vi "XYZ stage handler_coMD.vi"() -> ()   [LabVIEW 2012]
doc: "SciScan 1.2 160622"
uses:
  <vilib>/Analysis/coordinate.llb/Euler Rotation Order.ctl
  <vilib>/Utility/VariantDataType/Type.ctl
  GFG/GFGnumericGet.vi
  GFG/GFGbooleanGet.vi
  <vilib>/Analysis/coordinate.llb/3D Cartesian Coordinate Rotation (Euler) (Scalar).vi
  GFG/GFGfpRefGet.vi
  GFG/GFG library.lvlib
  <vilib>/Analysis/NI_AALPro.lvlib
  <vilib>/Utility/VariantDataType/VariantType.lvlib
panel:
  out "error out 2":errorcluster
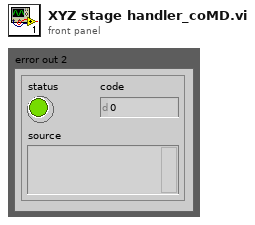
[diagram p1: front panel]
types:
  T1 = enum16{"none", "quit", "Press", "Long Press", "Long Press finished", "Short Press finished"}
  T2 = cluster{"WaveformChartRef":refnum<vi>, "DigitalRef":refnum<vi>, "ArrayRef":refnum<vi>, "TabControlRef":refnum<vi>, "EnumRef":refnum<vi>, "RingRef":refnum<vi>, "BooleanRef":refnum<vi>, "KnobRef":refnum<vi>, "SlideRef":refnum<vi>, "PathRef":refnum<vi>, "StringRef":refnum<vi>, "ComboBox":refnum<vi>, "WaveformGraphRef":refnum<vi>}
  T3 = cluster{"Xoffset":dbl, "Yoffset":dbl, "Zoffset":dbl}
  T4 = cluster{"moveXabs":dbl, "moveYabs":dbl, "moveZabs":dbl}
  T5 = cluster{"new pos X":dbl, "new pos Y":dbl, "new pos Z":dbl}
  T6 = typedef "NI_AALPro.lvlib/Euler Rotation Order.ctl" = u16
  T7 = cluster{"Numeric":dbl, "Numeric":dbl, "Numeric":dbl}
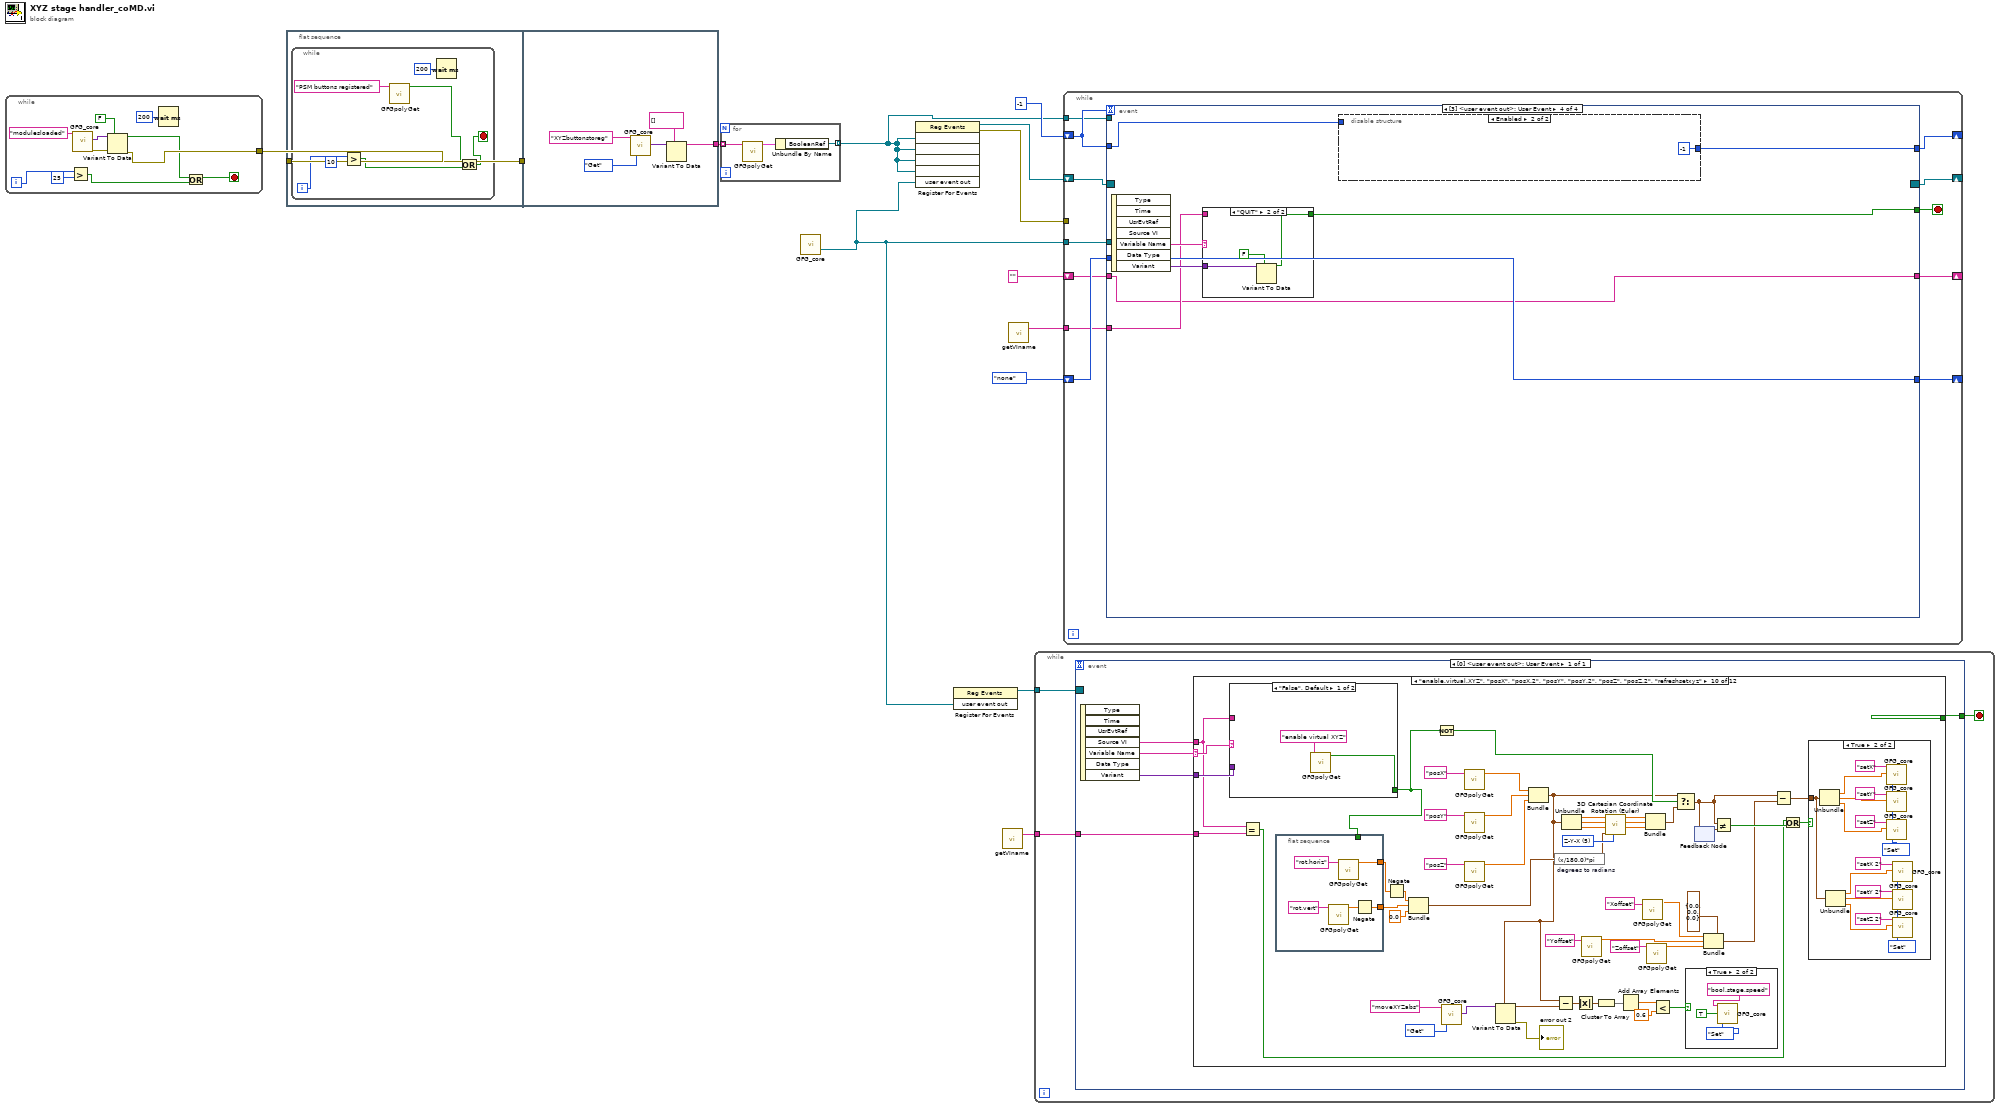
[diagram p0: block diagram]
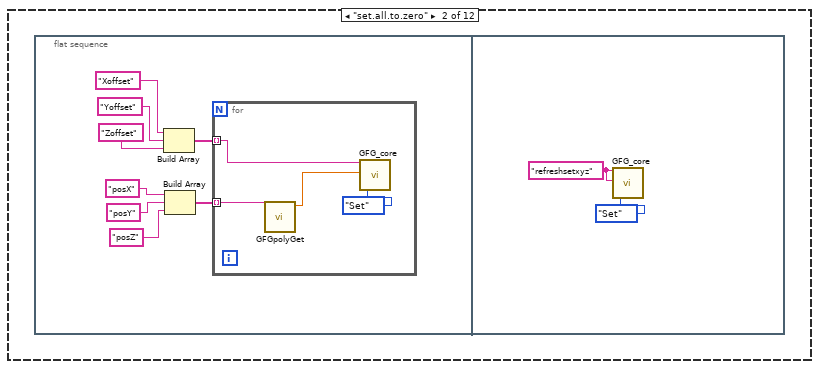
[diagram p3: hidden frame]
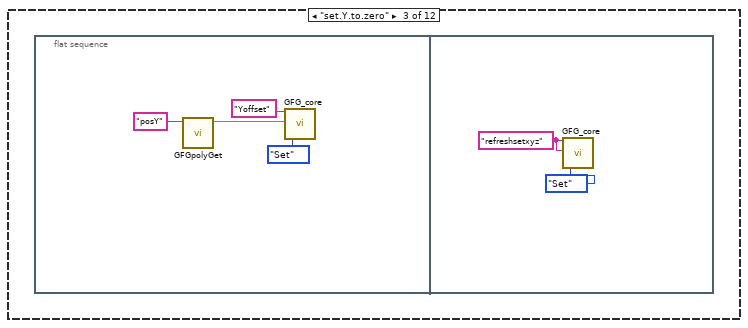
[diagram p4: hidden frame]
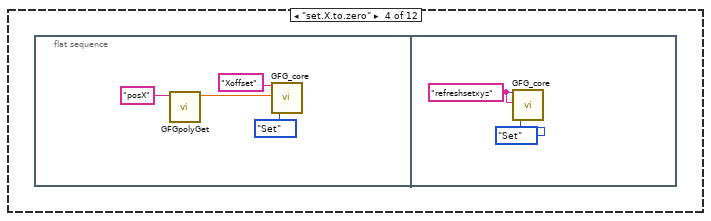
[diagram p5: hidden frame]
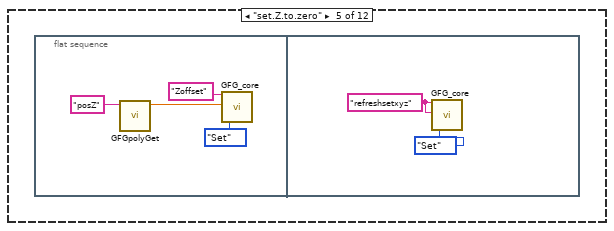
[diagram p6: hidden frame]
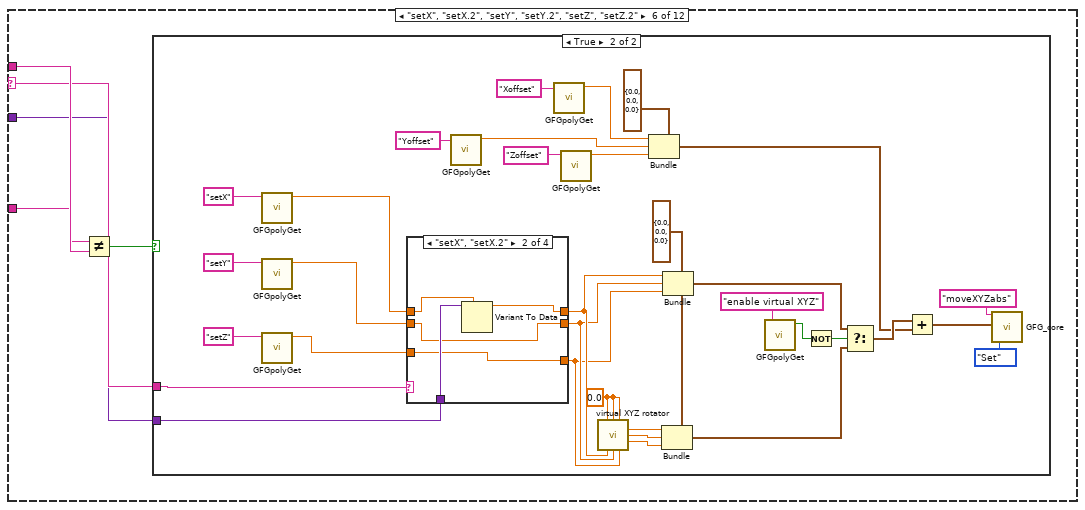
[diagram p7: hidden frame]
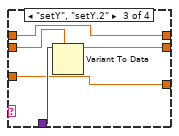
[diagram p10: hidden frame]
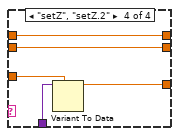
[diagram p11: hidden frame]
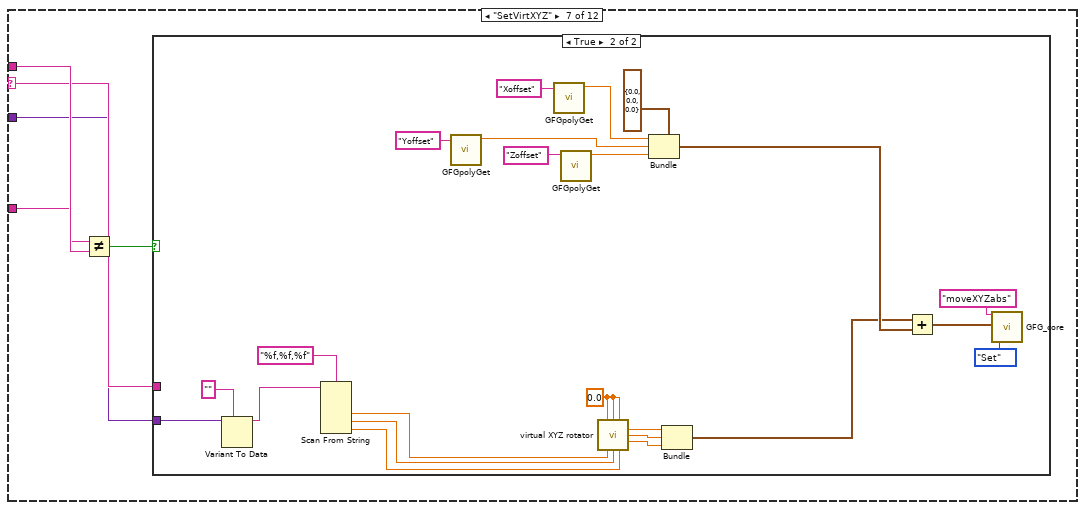
[diagram p12: hidden frame]
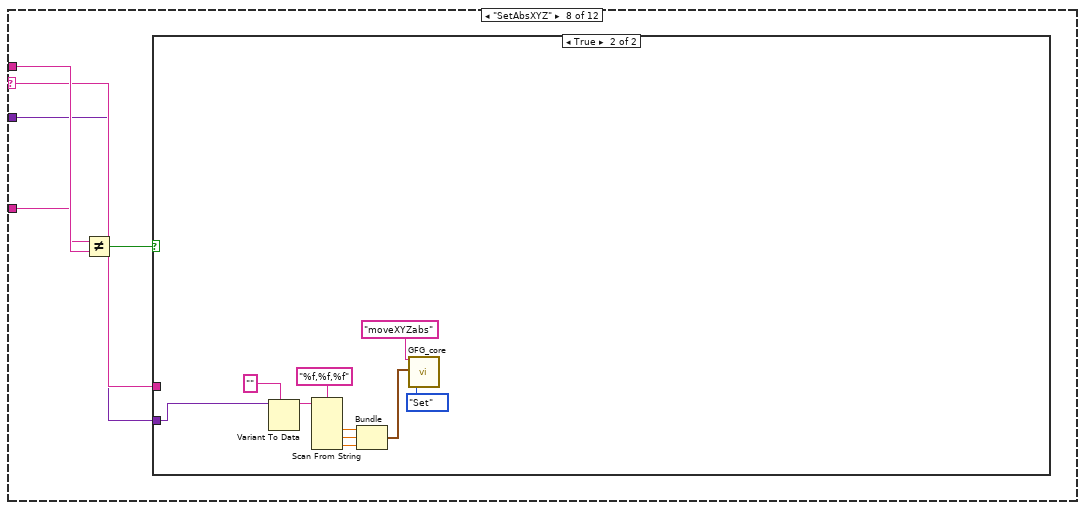
[diagram p14: hidden frame]
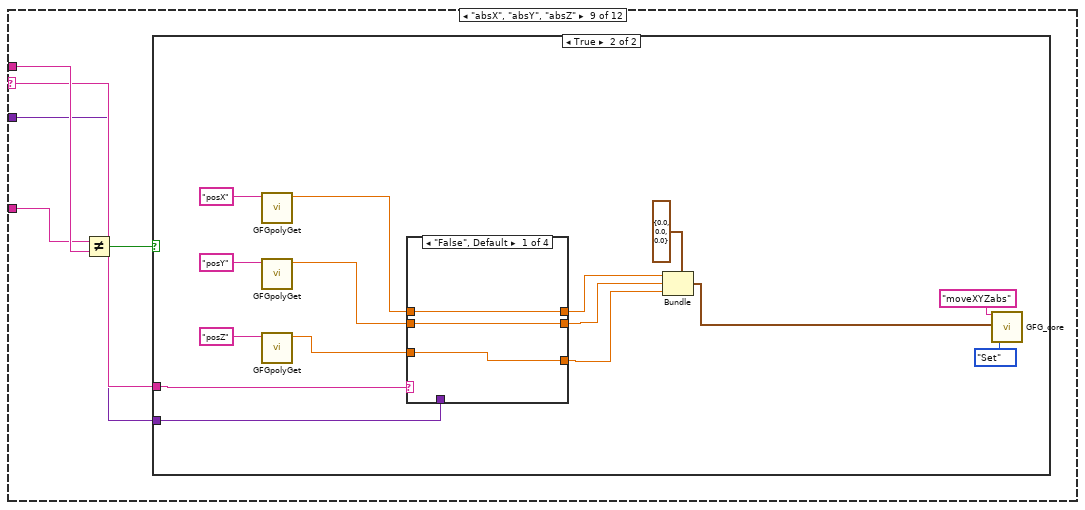
[diagram p16: hidden frame]
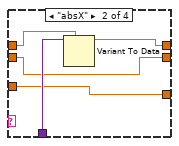
[diagram p18: hidden frame]
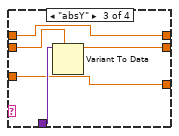
[diagram p19: hidden frame]
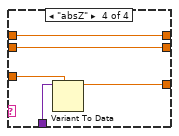
[diagram p20: hidden frame]
diagram:
  n1 = while {
    tunnel: [w19] -> w6
    i -> [w16]
    stop <- w17 stop-if-true
    n2 = Greater?(x=w16, y=25) -> (0:w14:bool)
    n3 = call "GFG_core.vi"("Variable Name in"="modulesloaded") -> ("Variant Out"=w20:variant, "error out"=w22:errorcluster)  [unwired: 12 in, 5 out]
    n4 = Variant To Data(error in=w22, type=FALSE, Variant=w20) -> (data=w18:bool, error out=w19:errorcluster)
    n5 = Wait (ms)(milliseconds to wait=u32 200) -> ()  [unwired: 1 out]
    n6 = Or(x=w18, y=w14) -> (x .or. y?=w17:bool)
  }
  n7 = flat-sequence {
    tunnel: w6 -> [w25]
    tunnel: [w25] -> w5
    tunnel: [w37] -> w7
    tunnel: w5 -> [_]
    frame #0 {
      n8 = while {
        i -> [w28]
        stop <- w26 stop-if-true
        n9 = Greater?(x=w28, y=10) -> (0:w30:bool)
        n10 = call-poly "GFGpolyGet.vi"("Variable Name in"="PSM buttons registered") -> ("Boolean Value OUT"=w27:bool)  [unwired: 9 in, 1 out]
        n11 = Wait (ms)(milliseconds to wait=u32 200) -> ()  [unwired: 1 out]
        n12 = Or(x=w27, y=w30) -> (x .or. y?=w26:bool)
      }
    }
    frame #1 {
      n13 = call "GFG_core.vi"("Variable Name in"="XYZbuttonstoreg", "Action"=enum16{"Init", "Set", "Get"}."Get") -> ("Variant Out"=w33:variant)  [unwired: 11 in, 6 out]
      n14 = Variant To Data(type=string[] [], Variant=w33) -> (data=w37:string[])  [unwired: 1 in, 1 out]
    }
  }
  n15 = for {
    tunnel: w7 -> [w39] mode=indexing
    tunnel: [w38] -> w4 mode=indexing
    n16 = call-poly "GFGpolyGet.vi"("Variable Name in"=w39) -> ("output cluster"=w40:T2)  [unwired: 9 in, 1 out]
    n17 = Unbundle By Name(w40) -> ("BooleanRef"=w38:refnum<vi>)
  }
  n18 = call "GFG_core.vi"() -> ("user event out"=w3:refnum<user-event>)  [unwired: 13 in, 6 out]
  n19 = register-events(w4, w4, w4, w4, w3) -> (reference out=w8:refnum<event-registration>, error out=w9:errorcluster)  [unwired: 2 in]
  n20 = register-events(w3) -> (reference out=w1:refnum<event-registration>)  [unwired: 2 in, 1 out]
  n21 = call "getVIname.vi"() -> ("VI name"=w2:string)  [unwired: 19 in]
  n22 = call "getVIname.vi"() -> ("VI name"=w10:string)  [unwired: 19 in]
  n23 = while {
    tunnel: w2 -> [w42]
    tunnel: w1 -> [w41]
    stop <- w43 stop-if-true
    n24 = event shown="[0] <user event out>: User Event" {
      selector: w41 -> [_]
      dyn-events: _ -> [_]
      timeout: _ -> [_]
      tunnel: [w46] -> w43
      tunnel: w42 -> [w44]
      event User Event {
        n25 = event-data() -> ("Source VI"=w45:string, "Variable Name"=w47:string, "Variant"=w48:variant)  [unwired: 1 in, 4 out]
        n26 = case shown="\"enable.virtual.XYZ\", \"posX\", \"posX.2\", \"posY\", \"posY.2\", \"posZ\", \"posZ.2\", \"refreshsetxyz\"" w47 {
          selector: w47 -> [_ _ _ _ _ w82 w138 w166 w181 w269 _ w308]
          tunnel: [_ _ _ _ _ _ _ _ _ _ w302 _] -> w46
          tunnel: w48 -> [_ _ _ _ _ w81 w137 w165 w180 w268 w304 _]
          tunnel: w45 -> [_ _ _ _ _ w85 w141 w169 w184 w218 _ _]
          tunnel: w44 -> [_ _ _ _ _ w84 w140 w168 w183 w220 _ _]
          frame "False", Default {
          }
          frame "set.all.to.zero" {
            n27 = flat-sequence {
              frame #0 {
                n28 = Build Array("Xoffset" ("Variable Name in"), "Yoffset" ("Variable Name in"), "Zoffset" ("Variable Name in")) -> (w56:string[])
                n29 = Build Array("posX" ("Variable Name in"), "posY" ("Variable Name in"), "posZ" ("Variable Name in")) -> (w52:string[])
                n30 = for {
                  tunnel: w52 -> [w59] mode=indexing
                  tunnel: w56 -> [w57] mode=indexing
                  n31 = call-poly "GFGpolyGet.vi"("Variable Name in"=w59) -> ("Numeric"=w58:dbl)  [unwired: 8 in, 2 out]
                  n32 = call "GFG_core.vi"("Variable Name in"=w57, "Variant in"=w58, "Action"=enum16{"Init", "Set", "Get"}."Set") -> ()  [unwired: 10 in, 7 out]
                }
              }
              frame #1 {
                w61 = "refreshsetxyz" ("Variable Name in")
                n33 = call "GFG_core.vi"("Variable Name in"=w61, "Variant in"=w61, "Action"=enum16{"Init", "Set", "Get"}."Set") -> ()  [unwired: 10 in, 7 out]
              }
            }
          }
          frame "set.Y.to.zero" {
            n34 = flat-sequence {
              frame #0 {
                n35 = call-poly "GFGpolyGet.vi"("Variable Name in"="posY") -> ("Numeric"=w64:dbl)  [unwired: 8 in, 2 out]
                n36 = call "GFG_core.vi"("Variable Name in"="Yoffset", "Variant in"=w64, "Action"=enum16{"Init", "Set", "Get"}."Set") -> ()  [unwired: 10 in, 7 out]
              }
              frame #1 {
                w67 = "refreshsetxyz" ("Variable Name in")
                n37 = call "GFG_core.vi"("Variable Name in"=w67, "Variant in"=w67, "Action"=enum16{"Init", "Set", "Get"}."Set") -> ()  [unwired: 10 in, 7 out]
              }
            }
          }
          frame "set.X.to.zero" {
            n38 = flat-sequence {
              frame #0 {
                n39 = call-poly "GFGpolyGet.vi"("Variable Name in"="posX") -> ("Numeric"=w70:dbl)  [unwired: 8 in, 2 out]
                n40 = call "GFG_core.vi"("Variable Name in"="Xoffset", "Variant in"=w70, "Action"=enum16{"Init", "Set", "Get"}."Set") -> ()  [unwired: 10 in, 7 out]
              }
              frame #1 {
                w73 = "refreshsetxyz" ("Variable Name in")
                n41 = call "GFG_core.vi"("Variable Name in"=w73, "Variant in"=w73, "Action"=enum16{"Init", "Set", "Get"}."Set") -> ()  [unwired: 10 in, 7 out]
              }
            }
          }
          frame "set.Z.to.zero" {
            n42 = flat-sequence {
              frame #0 {
                n43 = call-poly "GFGpolyGet.vi"("Variable Name in"="posZ") -> ("Numeric"=w76:dbl)  [unwired: 8 in, 2 out]
                n44 = call "GFG_core.vi"("Variable Name in"="Zoffset", "Variant in"=w76, "Action"=enum16{"Init", "Set", "Get"}."Set") -> ()  [unwired: 10 in, 7 out]
              }
              frame #1 {
                w79 = "refreshsetxyz" ("Variable Name in")
                n45 = call "GFG_core.vi"("Variable Name in"=w79, "Variant in"=w79, "Action"=enum16{"Init", "Set", "Get"}."Set") -> ()  [unwired: 10 in, 7 out]
              }
            }
          }
          frame "setX", "setX.2", "setY", "setY.2", "setZ", "setZ.2" {
            n46 = Not Equal?(x=w84, y=w85) -> (x != y?=w83:bool)
            n47 = case shown="True" w83 {
              tunnel: w82 -> [_ w112]
              tunnel: w81 -> [_ w111]
              frame False {
              }
              frame True {
                w101 = 0.0 ("current pos X")
                w106 = T4 {"moveXabs"=0.0, "moveYabs"=0.0, "moveZabs"=0.0} ("output cluster")
                n48 = call-poly "GFGpolyGet.vi"("Variable Name in"="setX") -> ("Numeric"=w117:dbl)  [unwired: 8 in, 2 out]
                n49 = call-poly "GFGpolyGet.vi"("Variable Name in"="setY") -> ("Numeric"=w116:dbl)  [unwired: 8 in, 2 out]
                n50 = call-poly "GFGpolyGet.vi"("Variable Name in"="setZ") -> ("Numeric"=w118:dbl)  [unwired: 8 in, 2 out]
                n51 = case shown="\"setX\", \"setX.2\"" w112 {
                  tunnel: w116 -> [w120 w125 w128 w134]
                  tunnel: w117 -> [w121 w122 w129 w135]
                  tunnel: w118 -> [w119 w123 w130 w133]
                  tunnel: w111 -> [_ w126 w131 w136]
                  tunnel: [w120 w125 w127 w134] -> w96
                  tunnel: [w121 w124 w129 w135] -> w97
                  tunnel: [w119 w123 w130 w132] -> w95
                  frame "False", Default {
                  }
                  frame "setX", "setX.2" {
                    n52 = Variant To Data(type=w122, Variant=w126) -> (data=w124:dbl)  [unwired: 1 in, 1 out]
                  }
                  frame "setY", "setY.2" {
                    n53 = Variant To Data(type=w128, Variant=w131) -> (data=w127:dbl)  [unwired: 1 in, 1 out]
                  }
                  frame "setZ", "setZ.2" {
                    n54 = Variant To Data(type=w133, Variant=w136) -> (data=w132:dbl)  [unwired: 1 in, 1 out]
                  }
                }
                n55 = call-poly "GFGpolyGet.vi"("Variable Name in"="Yoffset") -> ("Numeric"=w88:dbl)  [unwired: 8 in, 2 out]
                n56 = call-poly "GFGpolyGet.vi"("Variable Name in"="Xoffset") -> ("Numeric"=w89:dbl)  [unwired: 8 in, 2 out]
                n57 = call-poly "GFGpolyGet.vi"("Variable Name in"="Zoffset") -> ("Numeric"=w87:dbl)  [unwired: 8 in, 2 out]
                n58 = call "virtual XYZ rotator.vi"("current pos X"=w101, "current pos Y"=w101, "current pos Z"=w101, "virtual X relative"=w97, "virtual Y relative"=w96, "virtual Z relative"=w95) -> ("new pos X"=w109:dbl, "new pos Y"=w108:dbl, "new pos Z"=w107:dbl)  [unwired: 7 in]
                n59 = Bundle(cluster=T3 {"Xoffset"=0.0, "Yoffset"=0.0, "Zoffset"=0.0} ("output cluster"), "Xoffset"=w89, "Yoffset"=w88, "Zoffset"=w87) -> (w86:T3)
                n60 = Bundle(cluster=w106, "moveXabs"=w109, "moveYabs"=w108, "moveZabs"=w107) -> (w104:T4)
                n61 = Bundle(cluster=w106, "moveXabs"=w97, "moveYabs"=w96, "moveZabs"=w95) -> (w105:T4)
                n62 = call-poly "GFGpolyGet.vi"("Variable Name in"="enable virtual XYZ") -> ("Boolean Value OUT"=w103:bool)  [unwired: 9 in, 1 out]
                n63 = Not(x=w103) -> (.not. x?=w102:bool)
                n64 = Select(t=w105, s=w102, f=w104) -> (s? t:f=w98:T4)
                n65 = Add(x=w98, y=w86) -> (x+y=w94:cluster{dbl, dbl, dbl})
                n66 = call "GFG_core.vi"("Variable Name in"="moveXYZabs", "Variant in"=w94, "Action"=enum16{"Init", "Set", "Get"}."Set") -> ()  [unwired: 10 in, 7 out]
              }
            }
          }
          frame "SetVirtXYZ" {
            n67 = Not Equal?(x=w140, y=w141) -> (x != y?=w139:bool)
            n68 = case shown="True" w139 {
              tunnel: w138 -> [_ _]
              tunnel: w137 -> [_ w149]
              frame False {
              }
              frame True {
                w161 = 0.0 ("current pos X")
                n69 = Variant To Data(type="", Variant=w149) -> (data=w146:string)  [unwired: 1 in, 1 out]
                n70 = Scan From String(format string="%f,%f,%f", input string=w146) -> (output 1=w144:dbl, output 2=w143:dbl, output 3=w142:dbl)  [unwired: 5 in, 3 out]
                n71 = call-poly "GFGpolyGet.vi"("Variable Name in"="Yoffset") -> ("Numeric"=w152:dbl)  [unwired: 8 in, 2 out]
                n72 = call-poly "GFGpolyGet.vi"("Variable Name in"="Xoffset") -> ("Numeric"=w153:dbl)  [unwired: 8 in, 2 out]
                n73 = call-poly "GFGpolyGet.vi"("Variable Name in"="Zoffset") -> ("Numeric"=w151:dbl)  [unwired: 8 in, 2 out]
                n74 = call "virtual XYZ rotator.vi"("current pos X"=w161, "current pos Y"=w161, "current pos Z"=w161, "virtual X relative"=w144, "virtual Y relative"=w143, "virtual Z relative"=w142) -> ("new pos X"=w164:dbl, "new pos Y"=w163:dbl, "new pos Z"=w162:dbl)  [unwired: 7 in]
                n75 = Bundle(cluster=T3 {"Xoffset"=0.0, "Yoffset"=0.0, "Zoffset"=0.0} ("output cluster"), "Xoffset"=w153, "Yoffset"=w152, "Zoffset"=w151) -> (w150:T3)
                n76 = Bundle("new pos X"=w164, "new pos Y"=w163, "new pos Z"=w162) -> (w145:T5)  [unwired: 1 in]
                n77 = Add(x=w145, y=w150) -> (x+y=w158:cluster{dbl, dbl, dbl})
                n78 = call "GFG_core.vi"("Variable Name in"="moveXYZabs", "Variant in"=w158, "Action"=enum16{"Init", "Set", "Get"}."Set") -> ()  [unwired: 10 in, 7 out]
              }
            }
          }
          frame "SetAbsXYZ" {
            n79 = Not Equal?(x=w168, y=w169) -> (x != y?=w167:bool)
            n80 = case shown="True" w167 {
              tunnel: w166 -> [_ _]
              tunnel: w165 -> [_ w177]
              frame False {
              }
              frame True {
                n81 = Variant To Data(type="", Variant=w177) -> (data=w174:string)  [unwired: 1 in, 1 out]
                n82 = Scan From String(format string="%f,%f,%f", input string=w174) -> (output 1=w172:dbl, output 2=w171:dbl, output 3=w170:dbl)  [unwired: 5 in, 3 out]
                n83 = Bundle(w172, w171, w170) -> (w173:cluster{dbl, dbl, dbl})  [unwired: 1 in]
                n84 = call "GFG_core.vi"("Variable Name in"="moveXYZabs", "Variant in"=w173, "Action"=enum16{"Init", "Set", "Get"}."Set") -> ()  [unwired: 10 in, 7 out]
              }
            }
          }
          frame "absX", "absY", "absZ" {
            n85 = Not Equal?(x=w183, y=w184) -> (x != y?=w182:bool)
            n86 = case shown="True" w182 {
              tunnel: w181 -> [_ w193]
              tunnel: w180 -> [_ w192]
              frame False {
              }
              frame True {
                n87 = call-poly "GFGpolyGet.vi"("Variable Name in"="posX") -> ("Numeric"=w198:dbl)  [unwired: 8 in, 2 out]
                n88 = call-poly "GFGpolyGet.vi"("Variable Name in"="posY") -> ("Numeric"=w197:dbl)  [unwired: 8 in, 2 out]
                n89 = call-poly "GFGpolyGet.vi"("Variable Name in"="posZ") -> ("Numeric"=w199:dbl)  [unwired: 8 in, 2 out]
                n90 = case shown="\"False\", Default" w193 {
                  tunnel: w197 -> [w201 w206 w209 w215]
                  tunnel: w198 -> [w202 w203 w210 w216]
                  tunnel: w199 -> [w200 w204 w211 w214]
                  tunnel: w192 -> [_ w207 w212 w217]
                  tunnel: [w201 w206 w208 w215] -> w187
                  tunnel: [w202 w205 w210 w216] -> w188
                  tunnel: [w200 w204 w211 w213] -> w186
                  frame "False", Default {
                  }
                  frame "absX" {
                    n91 = Variant To Data(type=w203, Variant=w207) -> (data=w205:dbl)  [unwired: 1 in, 1 out]
                  }
                  frame "absY" {
                    n92 = Variant To Data(type=w209, Variant=w212) -> (data=w208:dbl)  [unwired: 1 in, 1 out]
                  }
                  frame "absZ" {
                    n93 = Variant To Data(type=w214, Variant=w217) -> (data=w213:dbl)  [unwired: 1 in, 1 out]
                  }
                }
                n94 = Bundle(cluster=T4 {"moveXabs"=0.0, "moveYabs"=0.0, "moveZabs"=0.0} ("output cluster"), "moveXabs"=w188, "moveYabs"=w187, "moveZabs"=w186) -> (w185:T4)
                n95 = call "GFG_core.vi"("Variable Name in"="moveXYZabs", "Variant in"=w185, "Action"=enum16{"Init", "Set", "Get"}."Set") -> ()  [unwired: 10 in, 7 out]
              }
            }
          }
          frame "enable.virtual.XYZ", "posX", "posX.2", "posY", "posY.2", "posZ", "posZ.2", "refreshsetxyz" {
            w259 = T6 5 items=["X-Y-Z", "X-Z-Y", "Y-X-Z", "Y-Z-X", "Z-X-Y", "Z-Y-X", "X-Y-X", "X-Z-X", "Y-X-Y", "Y-Z-Y", "Z-X-Z", "Z-Y-Z"] ("rotation order")
            n96 = case shown="\"False\", Default" w269 {
              tunnel: w268 -> [_ w301]
              tunnel: [w293 w299] -> w232
              tunnel: w218 -> [_ w298]
              frame "False", Default {
                n97 = call-poly "GFGpolyGet.vi"("Variable Name in"="enable virtual XYZ") -> ("Boolean Value OUT"=w293:bool)  [unwired: 9 in, 1 out]
              }
              frame "enable.virtual.XYZ" {
                n98 = Variant To Data(type=TRUE, Variant=w301) -> (data=w299:bool)  [unwired: 1 in, 1 out]
                n99 = Equal?(x="fp button handler_crMD.vi", y=w298) -> (x = y?=w295:bool)
                n100 = And(x=w295, y=w299) -> (x .and. y?=w296:bool)
                n101 = case shown="True" w296 {
                  frame False {
                  }
                  frame True {
                    n102 = call "set virtual Z rotation values.vi"() -> ()  [unwired: 12 in]
                  }
                }
              }
            }
            n103 = Equal?(x=w218, y=w220) -> (x = y?=w219:bool)
            n104 = flat-sequence {
              tunnel: [w274] -> w262
              tunnel: [w272] -> w260
              tunnel: w232 -> [_]
              frame #0 {
                n105 = call-poly "GFGpolyGet.vi"("Variable Name in"="rot.vert") -> ("Numeric"=w273:dbl)  [unwired: 8 in, 2 out]
                n106 = call-poly "GFGpolyGet.vi"("Variable Name in"="rot.horiz") -> ("Numeric"=w272:dbl)  [unwired: 8 in, 2 out]
                n107 = Negate(x=w273) -> (-x=w274:dbl)
              }
            }
            n108 = Negate(x=w260) -> (-x=w261:dbl)
            n109 = Bundle(w261, w262, "phi"=0.0) -> (w264:cluster{dbl, dbl, "phi":dbl})  [unwired: 1 in]
            n110 = Not(x=w232) -> (.not. x?=w248:bool)
            n111 = call "GFG_core.vi"("Variable Name in"="moveXYZabs", "Action"=enum16{"Init", "Set", "Get", "Clear"}."Get") -> ("Variant Out"=w243:variant)  [unwired: 11 in, 6 out]
            n112 = call-poly "GFGpolyGet.vi"("Variable Name in"="posX") -> ("Numeric"=w257:dbl)  [unwired: 8 in, 2 out]
            n113 = call-poly "GFGpolyGet.vi"("Variable Name in"="posY") -> ("Numeric"=w256:dbl)  [unwired: 8 in, 2 out]
            n114 = call-poly "GFGpolyGet.vi"("Variable Name in"="posZ") -> ("Numeric"=w255:dbl)  [unwired: 8 in, 2 out]
            n115 = Bundle("Numeric"=w257, "Numeric"=w256, "Numeric"=w255) -> (w240:T7)  [unwired: 1 in]
            n116 = Variant To Data(type=w240, Variant=w243) -> (data=w241:T7, error out=→"error out 2":errorcluster)  [unwired: 1 in]
            n117 = expression code="(x/180.0)*pi" "degrees to radians"(w264) -> (w258:cluster{dbl, dbl, "phi":dbl})
            n118 = Subtract(x=w240, y=w241) -> (x-y=w239:T7)
            n119 = Unbundle(w240) -> ("Numeric"=w254:dbl, "Numeric"=w253:dbl, "Numeric"=w252:dbl)
            n120 = Absolute Value(x=w239) -> (abs(x)=w238:T7)
            n121 = call-poly "GFGpolyGet.vi"("Variable Name in"="Yoffset") -> ("Numeric"=w226:dbl)  [unwired: 8 in, 2 out]
            n122 = Cluster To Array(cluster=w238) -> (array=w237:dbl[])
            n123 = call-poly <vilib>:"3D Cartesian Coordinate Rotation (Euler).vi"("rotation order"=w259, "Euler Angles"=w258, "z"=w252, "y"=w253, "x"=w254) -> ("z out"=w249:dbl, "y out"=w250:dbl, "x out"=w251:dbl)  [unwired: 3 in, 1 out]
            n124 = Add Array Elements(numeric array=w237) -> (sum=w236:dbl)
            n125 = call-poly "GFGpolyGet.vi"("Variable Name in"="Xoffset") -> ("Numeric"=w227:dbl)  [unwired: 8 in, 2 out]
            n126 = Bundle("x out"=w251, "y out"=w250, "z out"=w249) -> (w247:cluster{"x out":dbl, "y out":dbl, "z out":dbl})  [unwired: 1 in]
            n127 = call-poly "GFGpolyGet.vi"("Variable Name in"="Zoffset") -> ("Numeric"=w225:dbl)  [unwired: 8 in, 2 out]
            n128 = Less?(x=w236, y=0.6) -> (x < y?=w234:bool)
            n129 = Select(t=w240, s=w248, f=w247) -> (s? t:f=w223:cluster{"x out":dbl, "y out":dbl, "z out":dbl})
            n130 = case shown="True" w234 {
              frame False {
              }
              frame True {
                n131 = call "GFG_core.vi"("Variable Name in"="bool.stage.speed", "Variant in"=TRUE ("Boolean"), "Action"=enum16{"Init", "Set", "Get"}."Set") -> ()  [unwired: 10 in, 7 out]
              }
            }
            n132 = feedback-in #1(w223) -> ()
            n133 = feedback #1() -> (w245:cluster{"x out":dbl, "y out":dbl, "z out":dbl})  [unwired: 1 in]
            n134 = Bundle(cluster=T3 {"Xoffset"=0.0, "Yoffset"=0.0, "Zoffset"=0.0} ("output cluster"), "Xoffset"=w227, "Yoffset"=w226, "Zoffset"=w225) -> (w222:T3)
            n135 = Not Equal?(x=w223, y=w245) -> (x != y?=w246:bool)
            n136 = Subtract(x=w223, y=w222) -> (x-y=w224:cluster{dbl, dbl, dbl})
            n137 = Or(x=w219, y=w246) -> (x .or. y?=w221:bool)
            n138 = case shown="True" w221 {
              tunnel: w224 -> [_ w278]
              frame False {
              }
              frame True {
                w282 = enum16{"Init", "Set", "Get"}."Set" ("Action")
                w289 = enum16{"Init", "Set", "Get"}."Set" ("Action")
                n139 = Unbundle(w278) -> (w288:dbl, w287:dbl, w286:dbl)
                n140 = Unbundle(w278) -> (w283:dbl, w284:dbl, w285:dbl)
                n141 = call "GFG_core.vi"("Variable Name in"="setX", "Variant in"=w288, "Action"=w289) -> ()  [unwired: 10 in, 7 out]
                n142 = call "GFG_core.vi"("Variable Name in"="setY", "Variant in"=w287, "Action"=w289) -> ()  [unwired: 10 in, 7 out]
                n143 = call "GFG_core.vi"("Variable Name in"="setZ", "Variant in"=w286, "Action"=w289) -> ()  [unwired: 10 in, 7 out]
                n144 = call "GFG_core.vi"("Variable Name in"="setX 2", "Variant in"=w283, "Action"=w282) -> ()  [unwired: 10 in, 7 out]
                n145 = call "GFG_core.vi"("Variable Name in"="setY 2", "Variant in"=w284, "Action"=w282) -> ()  [unwired: 10 in, 7 out]
                n146 = call "GFG_core.vi"("Variable Name in"="setZ 2", "Variant in"=w285, "Action"=w282) -> ()  [unwired: 10 in, 7 out]
              }
            }
          }
          frame "QUIT" {
            n147 = Variant To Data(type=FALSE ("NewVal"), Variant=w304) -> (data=w302:bool)  [unwired: 1 in, 1 out]
          }
          frame "set.stage.speed" {
            n148 = call-poly "GFGpolyGet.vi"("Variable Name in"=w308) -> ("output cluster"=w307:T2)  [unwired: 9 in, 1 out]
            n149 = Unbundle By Name(w307) -> ("BooleanRef"=w306:refnum<vi>)
            n150 = property class="Bool"(reference=w306, "Value"=FALSE) -> ()  [unwired: 1 in, 2 out]
            n151 = call "set stage speeds.vi"() -> ()  [unwired: 12 in]
          }
        }
      }
    }
  }
  n152 = while {
    shift-right: [w318] -> _
    shift-left: -1 -> [w319]
    shift-right: [w316] -> _
    shift-left: T1."none" ("Enum") -> [w317]
    shift-right: [w315] -> _
    shift-left: "" ("Label.Text") -> [w314]
    tunnel: w3 -> [w313]
    tunnel: w10 -> [w311]
    tunnel: w9 -> [_]
    tunnel: w4 -> [w310]
    shift-right: [w309] -> _
    shift-left: w8 -> [w312]
    stop <- w320 stop-if-true
    n153 = event shown="[3] <user event out>: User Event" {
      selector: w312 -> [w321 w477 w495 _]
      dyn-events: [w321 w475 w492 _] -> w309
      timeout: w319 -> [_ _ _ _]
      tunnel: [_ _ _ w671] -> w320
      tunnel: w319 -> [_ _ _ w667]
      tunnel: [-1 w472 -1 w666] -> w318
      tunnel: w317 -> [_ _ w500 w670]
      tunnel: [T1."Long Press" ("Enum") T1."Press" ("Enum") w496 w670] -> w316
      tunnel: [w326 w480 w497 w668] -> w315
      tunnel: w314 -> [w326 _ w497 w668]
      tunnel: w313 -> [_ _ w493 _]
      tunnel: w311 -> [_ _ _ w669]
      tunnel: w310 -> [_ w476 w494 _]
      event Timeout {
        n154 = event-data() -> ()  [unwired: 1 in, 2 out]
        n155 = case shown="\"X LEFT\", \"X LEFT 2\"" w326 {
          tunnel: [w329 w339 w361 w387 w409 w433 w455] -> w322
          tunnel: 50000.0 ("-x") -> [_ w334 w357 w379 w402 w424 w447]
          frame "False", Default {
            n156 = call "GFG_core.vi"("Variable Name in"="moveXYZabs", "Action"=enum16{"Init", "Set", "Get"}."Get") -> ("Variant Out"=w331:variant)  [unwired: 11 in, 6 out]
            n157 = Variant To Data(type=T4 {"moveXabs"=0.0, "moveYabs"=0.0, "moveZabs"=0.0} ("output cluster"), Variant=w331) -> (data=w329:T4)  [unwired: 1 in, 1 out]
          }
          frame "Z UP", "Z UP 2" {
            w342 = T4 {"moveXabs"=0.0, "moveYabs"=0.0, "moveZabs"=0.0} ("output cluster")
            n158 = call-poly "GFGpolyGet.vi"("Variable Name in"="posZ") -> ("Numeric"=w346:dbl)  [unwired: 8 in, 2 out]
            n159 = call-poly "GFGpolyGet.vi"("Variable Name in"="posY") -> ("Numeric"=w347:dbl)  [unwired: 8 in, 2 out]
            n160 = call-poly "GFGpolyGet.vi"("Variable Name in"="posX") -> ("Numeric"=w348:dbl)  [unwired: 8 in, 2 out]
            n161 = call-poly "GFGpolyGet.vi"("Variable Name in"="reverse z") -> ("Boolean Value OUT"=w354:bool)  [unwired: 9 in, 1 out]
            n162 = Negate(x=w334) -> (-x=w355:dbl)
            n163 = Select(t=w334, s=w354, f=w355) -> (s? t:f=w336:dbl)
            n164 = Negate(x=w336) -> (-x=w335:dbl)
            n165 = call "virtual XYZ rotator.vi"("current pos X"=w348, "current pos Y"=w347, "current pos Z"=w346, "virtual Z relative"=w335) -> ("new pos X"=w345:dbl, "new pos Y"=w344:dbl, "new pos Z"=w343:dbl)  [unwired: 9 in]
            n166 = Add(x=w346, y=w335) -> (x+y=w350:dbl)
            n167 = Bundle(cluster=w342, "moveXabs"=w345, "moveYabs"=w344, "moveZabs"=w343) -> (w340:T4)
            n168 = Bundle(cluster=w342, "moveXabs"=w348, "moveYabs"=w347, "moveZabs"=w350) -> (w341:T4)
            n169 = call-poly "GFGpolyGet.vi"("Variable Name in"="enable virtual XYZ") -> ("Boolean Value OUT"=w338:bool)  [unwired: 9 in, 1 out]
            n170 = Not(x=w338) -> (.not. x?=w337:bool)
            n171 = Select(t=w341, s=w337, f=w340) -> (s? t:f=w339:T4)
          }
          frame "Z DOWN", "Z DOWN 2" {
            w364 = T4 {"moveXabs"=0.0, "moveYabs"=0.0, "moveZabs"=0.0} ("output cluster")
            n172 = call-poly "GFGpolyGet.vi"("Variable Name in"="posZ") -> ("Numeric"=w368:dbl)  [unwired: 8 in, 2 out]
            n173 = call-poly "GFGpolyGet.vi"("Variable Name in"="posY") -> ("Numeric"=w369:dbl)  [unwired: 8 in, 2 out]
            n174 = call-poly "GFGpolyGet.vi"("Variable Name in"="posX") -> ("Numeric"=w370:dbl)  [unwired: 8 in, 2 out]
            n175 = call-poly "GFGpolyGet.vi"("Variable Name in"="reverse z") -> ("Boolean Value OUT"=w376:bool)  [unwired: 9 in, 1 out]
            n176 = Negate(x=w357) -> (-x=w377:dbl)
            n177 = Select(t=w357, s=w376, f=w377) -> (s? t:f=w358:dbl)
            n178 = call "virtual XYZ rotator.vi"("current pos X"=w370, "current pos Y"=w369, "current pos Z"=w368, "virtual Z relative"=w358) -> ("new pos X"=w367:dbl, "new pos Y"=w366:dbl, "new pos Z"=w365:dbl)  [unwired: 9 in]
            n179 = Add(x=w368, y=w358) -> (x+y=w372:dbl)
            n180 = Bundle(cluster=w364, "moveXabs"=w367, "moveYabs"=w366, "moveZabs"=w365) -> (w362:T4)
            n181 = Bundle(cluster=w364, "moveXabs"=w370, "moveYabs"=w369, "moveZabs"=w372) -> (w363:T4)
            n182 = call-poly "GFGpolyGet.vi"("Variable Name in"="enable virtual XYZ") -> ("Boolean Value OUT"=w360:bool)  [unwired: 9 in, 1 out]
            n183 = Not(x=w360) -> (.not. x?=w359:bool)
            n184 = Select(t=w363, s=w359, f=w362) -> (s? t:f=w361:T4)
          }
          frame "Y UP", "Y UP 2" {
            w390 = T4 {"moveXabs"=0.0, "moveYabs"=0.0, "moveZabs"=0.0} ("output cluster")
            n185 = call-poly "GFGpolyGet.vi"("Variable Name in"="posZ") -> ("Numeric"=w381:dbl)  [unwired: 8 in, 2 out]
            n186 = call-poly "GFGpolyGet.vi"("Variable Name in"="posY") -> ("Numeric"=w383:dbl)  [unwired: 8 in, 2 out]
            n187 = call-poly "GFGpolyGet.vi"("Variable Name in"="posX") -> ("Numeric"=w394:dbl)  [unwired: 8 in, 2 out]
            n188 = call-poly "GFGpolyGet.vi"("Variable Name in"="reverse y") -> ("Boolean Value OUT"=w399:bool)  [unwired: 9 in, 1 out]
            n189 = Negate(x=w379) -> (-x=w400:dbl)
            n190 = Select(t=w379, s=w399, f=w400) -> (s? t:f=w384:dbl)
            n191 = Negate(x=w384) -> (-x=w380:dbl)
            n192 = call "virtual XYZ rotator.vi"("current pos X"=w394, "current pos Y"=w383, "current pos Z"=w381, "virtual Y relative"=w380) -> ("new pos X"=w393:dbl, "new pos Y"=w392:dbl, "new pos Z"=w391:dbl)  [unwired: 9 in]
            n193 = Add(x=w383, y=w380) -> (x+y=w382:dbl)
            n194 = Bundle(cluster=w390, "moveXabs"=w393, "moveYabs"=w392, "moveZabs"=w391) -> (w388:T4)
            n195 = Bundle(cluster=w390, "moveXabs"=w394, "moveYabs"=w382, "moveZabs"=w381) -> (w389:T4)
            n196 = call-poly "GFGpolyGet.vi"("Variable Name in"="enable virtual XYZ") -> ("Boolean Value OUT"=w386:bool)  [unwired: 9 in, 1 out]
            n197 = Not(x=w386) -> (.not. x?=w385:bool)
            n198 = Select(t=w389, s=w385, f=w388) -> (s? t:f=w387:T4)
          }
          frame "Y DOWN", "Y DOWN 2" {
            w412 = T4 {"moveXabs"=0.0, "moveYabs"=0.0, "moveZabs"=0.0} ("output cluster")
            n199 = call-poly "GFGpolyGet.vi"("Variable Name in"="posZ") -> ("Numeric"=w404:dbl)  [unwired: 8 in, 2 out]
            n200 = call-poly "GFGpolyGet.vi"("Variable Name in"="posY") -> ("Numeric"=w406:dbl)  [unwired: 8 in, 2 out]
            n201 = call-poly "GFGpolyGet.vi"("Variable Name in"="posX") -> ("Numeric"=w416:dbl)  [unwired: 8 in, 2 out]
            n202 = call-poly "GFGpolyGet.vi"("Variable Name in"="reverse y") -> ("Boolean Value OUT"=w421:bool)  [unwired: 9 in, 1 out]
            n203 = Negate(x=w402) -> (-x=w422:dbl)
            n204 = Select(t=w402, s=w421, f=w422) -> (s? t:f=w403:dbl)
            n205 = call "virtual XYZ rotator.vi"("current pos X"=w416, "current pos Y"=w406, "current pos Z"=w404, "virtual Y relative"=w403) -> ("new pos X"=w415:dbl, "new pos Y"=w414:dbl, "new pos Z"=w413:dbl)  [unwired: 9 in]
            n206 = Add(x=w406, y=w403) -> (x+y=w405:dbl)
            n207 = Bundle(cluster=w412, "moveXabs"=w415, "moveYabs"=w414, "moveZabs"=w413) -> (w410:T4)
            n208 = Bundle(cluster=w412, "moveXabs"=w416, "moveYabs"=w405, "moveZabs"=w404) -> (w411:T4)
            n209 = call-poly "GFGpolyGet.vi"("Variable Name in"="enable virtual XYZ") -> ("Boolean Value OUT"=w408:bool)  [unwired: 9 in, 1 out]
            n210 = Not(x=w408) -> (.not. x?=w407:bool)
            n211 = Select(t=w411, s=w407, f=w410) -> (s? t:f=w409:T4)
          }
          frame "X LEFT", "X LEFT 2" {
            w436 = T4 {"moveXabs"=0.0, "moveYabs"=0.0, "moveZabs"=0.0} ("output cluster")
            n212 = call-poly "GFGpolyGet.vi"("Variable Name in"="posZ") -> ("Numeric"=w430:dbl)  [unwired: 8 in, 2 out]
            n213 = call-poly "GFGpolyGet.vi"("Variable Name in"="posY") -> ("Numeric"=w427:dbl)  [unwired: 8 in, 2 out]
            n214 = call-poly "GFGpolyGet.vi"("Variable Name in"="posX") -> ("Numeric"=w429:dbl)  [unwired: 8 in, 2 out]
            n215 = call-poly "GFGpolyGet.vi"("Variable Name in"="reverse x") -> ("Boolean Value OUT"=w444:bool)  [unwired: 9 in, 1 out]
            n216 = Negate(x=w424) -> (-x=w445:dbl)
            n217 = Select(t=w424, s=w444, f=w445) -> (s? t:f=w426:dbl)
            n218 = Negate(x=w426) -> (-x=w425:dbl)
            n219 = call "virtual XYZ rotator.vi"("current pos X"=w429, "current pos Y"=w427, "current pos Z"=w430, "virtual X relative"=w425) -> ("new pos X"=w439:dbl, "new pos Y"=w438:dbl, "new pos Z"=w437:dbl)  [unwired: 9 in]
            n220 = Add(x=w429, y=w425) -> (x+y=w428:dbl)
            n221 = Bundle(cluster=w436, "moveXabs"=w439, "moveYabs"=w438, "moveZabs"=w437) -> (w434:T4)
            n222 = Bundle(cluster=w436, "moveXabs"=w428, "moveYabs"=w427, "moveZabs"=w430) -> (w435:T4)
            n223 = call-poly "GFGpolyGet.vi"("Variable Name in"="enable virtual XYZ") -> ("Boolean Value OUT"=w432:bool)  [unwired: 9 in, 1 out]
            n224 = Not(x=w432) -> (.not. x?=w431:bool)
            n225 = Select(t=w435, s=w431, f=w434) -> (s? t:f=w433:T4)
          }
          frame "X RIGHT", "X RIGHT 2" {
            w458 = T4 {"moveXabs"=0.0, "moveYabs"=0.0, "moveZabs"=0.0} ("output cluster")
            n226 = call-poly "GFGpolyGet.vi"("Variable Name in"="posZ") -> ("Numeric"=w452:dbl)  [unwired: 8 in, 2 out]
            n227 = call-poly "GFGpolyGet.vi"("Variable Name in"="posY") -> ("Numeric"=w449:dbl)  [unwired: 8 in, 2 out]
            n228 = call-poly "GFGpolyGet.vi"("Variable Name in"="posX") -> ("Numeric"=w451:dbl)  [unwired: 8 in, 2 out]
            n229 = call-poly "GFGpolyGet.vi"("Variable Name in"="reverse x") -> ("Boolean Value OUT"=w466:bool)  [unwired: 9 in, 1 out]
            n230 = Negate(x=w447) -> (-x=w467:dbl)
            n231 = Select(t=w447, s=w466, f=w467) -> (s? t:f=w448:dbl)
            n232 = call "virtual XYZ rotator.vi"("current pos X"=w451, "current pos Y"=w449, "current pos Z"=w452, "virtual X relative"=w448) -> ("new pos X"=w461:dbl, "new pos Y"=w460:dbl, "new pos Z"=w459:dbl)  [unwired: 9 in]
            n233 = Add(x=w451, y=w448) -> (x+y=w450:dbl)
            n234 = Bundle(cluster=w458, "moveXabs"=w461, "moveYabs"=w460, "moveZabs"=w459) -> (w456:T4)
            n235 = Bundle(cluster=w458, "moveXabs"=w450, "moveYabs"=w449, "moveZabs"=w452) -> (w457:T4)
            n236 = call-poly "GFGpolyGet.vi"("Variable Name in"="enable virtual XYZ") -> ("Boolean Value OUT"=w454:bool)  [unwired: 9 in, 1 out]
            n237 = Not(x=w454) -> (.not. x?=w453:bool)
            n238 = Select(t=w457, s=w453, f=w456) -> (s? t:f=w455:T4)
          }
        }
        n239 = call "GFG_core.vi"("Variable Name in"="moveXYZabs", "Variant in"=w322, "Action"=enum16{"Init", "Set", "Get"}."Set") -> ()  [unwired: 10 in, 7 out]
      }
      event Mouse Down {
        n240 = event-data() -> ("CtlRef"=w479:refnum<vi>)  [unwired: 1 in, 5 out]
        n241 = disable-structure shown="Enabled" {
          disable-tunnel: w477 -> [w486 w487]
          disable-tunnel: w476 -> [w485 _]
          disable-tunnel: [w484 w487] -> w475
          disable-tunnel: [w483 _] -> w474
          frame Enabled {
            n242 = register-events(reference=w486, w485, w485, w485, w485, refnum<user-event> refnum ("user event out")) -> (reference out=w484:refnum<event-registration>, error out=w483:errorcluster)  [unwired: 1 in]
          }
          frame Disabled {
          }
        }
        n243 = property class="Bool"(reference=w479, "Value"=TRUE) -> ()  [unwired: 1 in, 2 out]
        n244 = property class="Bool"(reference=w479) -> ("Label.Text"=w480:string)  [unwired: 1 in, 2 out]
        n245 = flat-sequence {
          tunnel: w474 -> [_]
          frame #0 {
            n246 = call "GFG_core.vi"("Variable Name in"="bool.stage.speed", "Variant in"=FALSE ("Boolean"), "Action"=enum16{"Init", "Set", "Get"}."Set") -> ()  [unwired: 10 in, 7 out]
          }
        }
        n247 = call-poly "GFGpolyGet.vi"("Variable Name in"="LP.enable") -> ("Boolean Value OUT"=w470:bool)  [unwired: 9 in, 1 out]
        n248 = Select(t=250, s=w470, f=-1) -> (s? t:f=w472:i32)
      }
      event Mouse Up; Mouse Leave {
        n249 = event-data() -> ("CtlRef"=w499:refnum<vi>)  [unwired: 1 in, 2 out]
        n250 = disable-structure shown="Enabled" {
          disable-tunnel: w495 -> [w506 w507]
          disable-tunnel: w494 -> [w505 _]
          disable-tunnel: w493 -> [w504 _]
          disable-tunnel: [w503 w507] -> w492
          disable-tunnel: [w502 _] -> w491
          frame Enabled {
            n251 = register-events(reference=w506, w505, w505, w505, w505, w504) -> (reference out=w503:refnum<event-registration>, error out=w502:errorcluster)  [unwired: 1 in]
          }
          frame Disabled {
          }
        }
        n252 = case shown="\"Press\"" w500 {
          selector: w500 -> [w508 _ _ w664 w665]
          tunnel: [w508 T1."Short Press finished" ("Enum") T1."Long Press finished" ("Enum") w664 w665] -> w496
          tunnel: w499 -> [_ _ _ _ _]
          tunnel: w497 -> [_ w512 _ _ _]
          tunnel: w491 -> [_ _ _ _ _]
          frame "none", Default {
          }
          frame "Press" {
            n253 = case shown="\"X LEFT\", \"X LEFT 2\"" w512 {
              tunnel: [w514 w523 w546 w573 w596 w621 w644] -> w509
              frame "False", Default {
                n254 = call "GFG_core.vi"("Variable Name in"="moveXYZabs", "Action"=enum16{"Init", "Set", "Get"}."Get") -> ("Variant Out"=w516:variant)  [unwired: 11 in, 6 out]
                n255 = Variant To Data(type=T4 {"moveXabs"=0.0, "moveYabs"=0.0, "moveZabs"=0.0} ("output cluster"), Variant=w516) -> (data=w514:T4)  [unwired: 1 in, 1 out]
              }
              frame "Z UP", "Z UP 2" {
                w526 = T4 {"moveXabs"=0.0, "moveYabs"=0.0, "moveZabs"=0.0} ("output cluster")
                n256 = call-poly "GFGpolyGet.vi"("Variable Name in"="posZ") -> ("Numeric"=w530:dbl)  [unwired: 8 in, 2 out]
                n257 = call-poly "GFGpolyGet.vi"("Variable Name in"="posY") -> ("Numeric"=w531:dbl)  [unwired: 8 in, 2 out]
                n258 = call-poly "GFGpolyGet.vi"("Variable Name in"="posX") -> ("Numeric"=w532:dbl)  [unwired: 8 in, 2 out]
                n259 = call-poly "GFGpolyGet.vi"("Variable Name in"="reverse z") -> ("Boolean Value OUT"=w538:bool)  [unwired: 9 in, 1 out]
                n260 = call-poly "GFGpolyGet.vi"("Variable Name in"="step.size.z") -> ("Numeric"=w539:dbl)  [unwired: 8 in, 2 out]
                n261 = Negate(x=w539) -> (-x=w540:dbl)
                n262 = Select(t=w539, s=w538, f=w540) -> (s? t:f=w520:dbl)
                n263 = Negate(x=w520) -> (-x=w519:dbl)
                n264 = call "virtual XYZ rotator.vi"("current pos X"=w532, "current pos Y"=w531, "current pos Z"=w530, "virtual Z relative"=w519) -> ("new pos X"=w529:dbl, "new pos Y"=w528:dbl, "new pos Z"=w527:dbl)  [unwired: 9 in]
                n265 = Add(x=w530, y=w519) -> (x+y=w534:dbl)
                n266 = Bundle(cluster=w526, "moveXabs"=w529, "moveYabs"=w528, "moveZabs"=w527) -> (w524:T4)
                n267 = Bundle(cluster=w526, "moveXabs"=w532, "moveYabs"=w531, "moveZabs"=w534) -> (w525:T4)
                n268 = call-poly "GFGpolyGet.vi"("Variable Name in"="enable virtual XYZ") -> ("Boolean Value OUT"=w522:bool)  [unwired: 9 in, 1 out]
                n269 = Not(x=w522) -> (.not. x?=w521:bool)
                n270 = Select(t=w525, s=w521, f=w524) -> (s? t:f=w523:T4)
              }
              frame "Z DOWN", "Z DOWN 2" {
                w549 = T4 {"moveXabs"=0.0, "moveYabs"=0.0, "moveZabs"=0.0} ("output cluster")
                n271 = call-poly "GFGpolyGet.vi"("Variable Name in"="posZ") -> ("Numeric"=w553:dbl)  [unwired: 8 in, 2 out]
                n272 = call-poly "GFGpolyGet.vi"("Variable Name in"="posY") -> ("Numeric"=w554:dbl)  [unwired: 8 in, 2 out]
                n273 = call-poly "GFGpolyGet.vi"("Variable Name in"="posX") -> ("Numeric"=w555:dbl)  [unwired: 8 in, 2 out]
                n274 = call-poly "GFGpolyGet.vi"("Variable Name in"="reverse z") -> ("Boolean Value OUT"=w561:bool)  [unwired: 9 in, 1 out]
                n275 = call-poly "GFGpolyGet.vi"("Variable Name in"="step.size.z") -> ("Numeric"=w562:dbl)  [unwired: 8 in, 2 out]
                n276 = Negate(x=w562) -> (-x=w563:dbl)
                n277 = Select(t=w562, s=w561, f=w563) -> (s? t:f=w543:dbl)
                n278 = call "virtual XYZ rotator.vi"("current pos X"=w555, "current pos Y"=w554, "current pos Z"=w553, "virtual Z relative"=w543) -> ("new pos X"=w552:dbl, "new pos Y"=w551:dbl, "new pos Z"=w550:dbl)  [unwired: 9 in]
                n279 = Add(x=w553, y=w543) -> (x+y=w557:dbl)
                n280 = Bundle(cluster=w549, "moveXabs"=w552, "moveYabs"=w551, "moveZabs"=w550) -> (w547:T4)
                n281 = Bundle(cluster=w549, "moveXabs"=w555, "moveYabs"=w554, "moveZabs"=w557) -> (w548:T4)
                n282 = call-poly "GFGpolyGet.vi"("Variable Name in"="enable virtual XYZ") -> ("Boolean Value OUT"=w545:bool)  [unwired: 9 in, 1 out]
                n283 = Not(x=w545) -> (.not. x?=w544:bool)
                n284 = Select(t=w548, s=w544, f=w547) -> (s? t:f=w546:T4)
              }
              frame "Y UP", "Y UP 2" {
                w576 = T4 {"moveXabs"=0.0, "moveYabs"=0.0, "moveZabs"=0.0} ("output cluster")
                n285 = call-poly "GFGpolyGet.vi"("Variable Name in"="posZ") -> ("Numeric"=w567:dbl)  [unwired: 8 in, 2 out]
                n286 = call-poly "GFGpolyGet.vi"("Variable Name in"="posY") -> ("Numeric"=w569:dbl)  [unwired: 8 in, 2 out]
                n287 = call-poly "GFGpolyGet.vi"("Variable Name in"="posX") -> ("Numeric"=w580:dbl)  [unwired: 8 in, 2 out]
                n288 = call-poly "GFGpolyGet.vi"("Variable Name in"="reverse y") -> ("Boolean Value OUT"=w585:bool)  [unwired: 9 in, 1 out]
                n289 = call-poly "GFGpolyGet.vi"("Variable Name in"="step.size.xy") -> ("Numeric"=w586:dbl)  [unwired: 8 in, 2 out]
                n290 = Negate(x=w586) -> (-x=w587:dbl)
                n291 = Select(t=w586, s=w585, f=w587) -> (s? t:f=w570:dbl)
                n292 = Negate(x=w570) -> (-x=w566:dbl)
                n293 = call "virtual XYZ rotator.vi"("current pos X"=w580, "current pos Y"=w569, "current pos Z"=w567, "virtual Y relative"=w566) -> ("new pos X"=w579:dbl, "new pos Y"=w578:dbl, "new pos Z"=w577:dbl)  [unwired: 9 in]
                n294 = Add(x=w569, y=w566) -> (x+y=w568:dbl)
                n295 = Bundle(cluster=w576, "moveXabs"=w579, "moveYabs"=w578, "moveZabs"=w577) -> (w574:T4)
                n296 = Bundle(cluster=w576, "moveXabs"=w580, "moveYabs"=w568, "moveZabs"=w567) -> (w575:T4)
                n297 = call-poly "GFGpolyGet.vi"("Variable Name in"="enable virtual XYZ") -> ("Boolean Value OUT"=w572:bool)  [unwired: 9 in, 1 out]
                n298 = Not(x=w572) -> (.not. x?=w571:bool)
                n299 = Select(t=w575, s=w571, f=w574) -> (s? t:f=w573:T4)
              }
              frame "Y DOWN", "Y DOWN 2" {
                w599 = T4 {"moveXabs"=0.0, "moveYabs"=0.0, "moveZabs"=0.0} ("output cluster")
                n300 = call-poly "GFGpolyGet.vi"("Variable Name in"="posZ") -> ("Numeric"=w591:dbl)  [unwired: 8 in, 2 out]
                n301 = call-poly "GFGpolyGet.vi"("Variable Name in"="posY") -> ("Numeric"=w593:dbl)  [unwired: 8 in, 2 out]
                n302 = call-poly "GFGpolyGet.vi"("Variable Name in"="posX") -> ("Numeric"=w603:dbl)  [unwired: 8 in, 2 out]
                n303 = call-poly "GFGpolyGet.vi"("Variable Name in"="reverse y") -> ("Boolean Value OUT"=w608:bool)  [unwired: 9 in, 1 out]
                n304 = call-poly "GFGpolyGet.vi"("Variable Name in"="step.size.xy") -> ("Numeric"=w609:dbl)  [unwired: 8 in, 2 out]
                n305 = Negate(x=w609) -> (-x=w610:dbl)
                n306 = Select(t=w609, s=w608, f=w610) -> (s? t:f=w590:dbl)
                n307 = call "virtual XYZ rotator.vi"("current pos X"=w603, "current pos Y"=w593, "current pos Z"=w591, "virtual Y relative"=w590) -> ("new pos X"=w602:dbl, "new pos Y"=w601:dbl, "new pos Z"=w600:dbl)  [unwired: 9 in]
                n308 = Add(x=w593, y=w590) -> (x+y=w592:dbl)
                n309 = Bundle(cluster=w599, "moveXabs"=w602, "moveYabs"=w601, "moveZabs"=w600) -> (w597:T4)
                n310 = Bundle(cluster=w599, "moveXabs"=w603, "moveYabs"=w592, "moveZabs"=w591) -> (w598:T4)
                n311 = call-poly "GFGpolyGet.vi"("Variable Name in"="enable virtual XYZ") -> ("Boolean Value OUT"=w595:bool)  [unwired: 9 in, 1 out]
                n312 = Not(x=w595) -> (.not. x?=w594:bool)
                n313 = Select(t=w598, s=w594, f=w597) -> (s? t:f=w596:T4)
              }
              frame "X LEFT", "X LEFT 2" {
                w624 = T4 {"moveXabs"=0.0, "moveYabs"=0.0, "moveZabs"=0.0} ("output cluster")
                n314 = call-poly "GFGpolyGet.vi"("Variable Name in"="reverse x") -> ("Boolean Value OUT"=w632:bool)  [unwired: 9 in, 1 out]
                n315 = call-poly "GFGpolyGet.vi"("Variable Name in"="step.size.xy") -> ("Numeric"=w633:dbl)  [unwired: 8 in, 2 out]
                n316 = Negate(x=w633) -> (-x=w634:dbl)
                n317 = call-poly "GFGpolyGet.vi"("Variable Name in"="posZ") -> ("Numeric"=w618:dbl)  [unwired: 8 in, 2 out]
                n318 = call-poly "GFGpolyGet.vi"("Variable Name in"="posY") -> ("Numeric"=w615:dbl)  [unwired: 8 in, 2 out]
                n319 = call-poly "GFGpolyGet.vi"("Variable Name in"="posX") -> ("Numeric"=w617:dbl)  [unwired: 8 in, 2 out]
                n320 = Select(t=w633, s=w632, f=w634) -> (s? t:f=w614:dbl)
                n321 = Negate(x=w614) -> (-x=w613:dbl)
                n322 = call "virtual XYZ rotator.vi"("current pos X"=w617, "current pos Y"=w615, "current pos Z"=w618, "virtual X relative"=w613) -> ("new pos X"=w627:dbl, "new pos Y"=w626:dbl, "new pos Z"=w625:dbl)  [unwired: 9 in]
                n323 = Add(x=w617, y=w613) -> (x+y=w616:dbl)
                n324 = Bundle(cluster=w624, "moveXabs"=w627, "moveYabs"=w626, "moveZabs"=w625) -> (w622:T4)
                n325 = Bundle(cluster=w624, "moveXabs"=w616, "moveYabs"=w615, "moveZabs"=w618) -> (w623:T4)
                n326 = call-poly "GFGpolyGet.vi"("Variable Name in"="enable virtual XYZ") -> ("Boolean Value OUT"=w620:bool)  [unwired: 9 in, 1 out]
                n327 = Not(x=w620) -> (.not. x?=w619:bool)
                n328 = Select(t=w623, s=w619, f=w622) -> (s? t:f=w621:T4)
              }
              frame "X RIGHT", "X RIGHT 2" {
                w647 = T4 {"moveXabs"=0.0, "moveYabs"=0.0, "moveZabs"=0.0} ("output cluster")
                n329 = call-poly "GFGpolyGet.vi"("Variable Name in"="posZ") -> ("Numeric"=w641:dbl)  [unwired: 8 in, 2 out]
                n330 = call-poly "GFGpolyGet.vi"("Variable Name in"="posY") -> ("Numeric"=w638:dbl)  [unwired: 8 in, 2 out]
                n331 = call-poly "GFGpolyGet.vi"("Variable Name in"="posX") -> ("Numeric"=w640:dbl)  [unwired: 8 in, 2 out]
                n332 = call-poly "GFGpolyGet.vi"("Variable Name in"="reverse x") -> ("Boolean Value OUT"=w655:bool)  [unwired: 9 in, 1 out]
                n333 = call-poly "GFGpolyGet.vi"("Variable Name in"="step.size.xy") -> ("Numeric"=w656:dbl)  [unwired: 8 in, 2 out]
                n334 = Negate(x=w656) -> (-x=w657:dbl)
                n335 = Select(t=w656, s=w655, f=w657) -> (s? t:f=w637:dbl)
                n336 = call "virtual XYZ rotator.vi"("current pos X"=w640, "current pos Y"=w638, "current pos Z"=w641, "virtual X relative"=w637) -> ("new pos X"=w650:dbl, "new pos Y"=w649:dbl, "new pos Z"=w648:dbl)  [unwired: 9 in]
                n337 = Add(x=w640, y=w637) -> (x+y=w639:dbl)
                n338 = Bundle(cluster=w647, "moveXabs"=w650, "moveYabs"=w649, "moveZabs"=w648) -> (w645:T4)
                n339 = Bundle(cluster=w647, "moveXabs"=w639, "moveYabs"=w638, "moveZabs"=w641) -> (w646:T4)
                n340 = call-poly "GFGpolyGet.vi"("Variable Name in"="enable virtual XYZ") -> ("Boolean Value OUT"=w643:bool)  [unwired: 9 in, 1 out]
                n341 = Not(x=w643) -> (.not. x?=w642:bool)
                n342 = Select(t=w646, s=w642, f=w645) -> (s? t:f=w644:T4)
              }
            }
            n343 = call "GFG_core.vi"("Variable Name in"="moveXYZabs", "Variant in"=w509, "Action"=enum16{"Init", "Set", "Get"}."Set") -> ()  [unwired: 10 in, 7 out]
          }
          frame "Long Press" {
            n344 = call "GFG_core.vi"("Variable Name in"="Stage.Stop", "Variant in"=TRUE, "Action"=enum16{"Init", "Set", "Get"}."Set") -> ()  [unwired: 10 in, 7 out]
          }
          frame "Long Press finished" {
          }
          frame "Short Press finished" {
          }
        }
        n345 = property class="Bool"(reference=w499, "Value"=FALSE) -> ()  [unwired: 1 in, 2 out]
      }
      event User Event {
        n346 = event-data() -> ("Variable Name"=w672:string, "Variant"=w673:variant)  [unwired: 1 in, 5 out]
        n347 = case shown="\"QUIT\"" w672 {
          tunnel: [_ w683] -> w671
          tunnel: w673 -> [_ w685]
          tunnel: w669 -> [_ _]
          frame "False", Default {
          }
          frame "QUIT" {
            n348 = Variant To Data(type=FALSE ("NewVal"), Variant=w685) -> (data=w683:bool)  [unwired: 1 in, 1 out]
          }
        }
        n349 = disable-structure shown="Enabled" {
          disable-tunnel: w667 -> [w676 _]
          disable-tunnel: [w675 -1] -> w666
          frame Disabled {
            # "Less than timeout preset?"
            # "Time Elapsed between user events"
            n350 = Tick Count (ms)() -> (millisecond timer value=w681:u32)
            n351 = feedback #2() -> (w680:u32)  [unwired: 1 in]
            n352 = feedback-in #2(w681) -> ()
            n353 = Subtract(x=w681, y=w680) -> (x-y=w679:u32)
            n354 = To Long Integer(number=w679) -> (32bit integer=w674:i32)
            n355 = Less?(x=w674, y=w676) -> (x < y?=w678:bool)
            n356 = Subtract(x=w676, y=w674) -> (x-y=w677:i32)
            n357 = Select(t=w677, s=w678, f=w676) -> (s? t:f=w675:i32)
          }
          frame Enabled {
          }
        }
      }
    }
  }
